vi "extract and prune to time range 3d.vi"(7 "prune?":bool=TRUE, 8 "error in (no error)":errorcluster, 9 "t0":dbl=-1.0, 10 "time range":dbl=-1.0, 11 "queue in":refnum<queue>) -> (0 "error out":errorcluster, 2 "extracted data":T1[](array[typedef]), 3 "queue out":refnum<queue>)   [LabVIEW 2017]
uses:
  typedefs/reading3.ctl
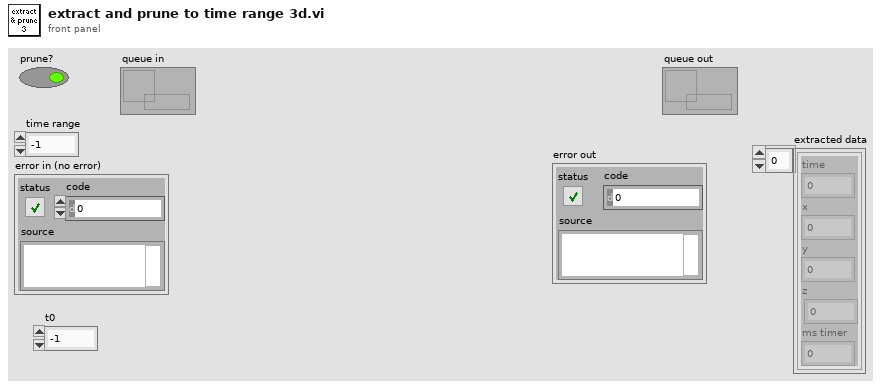
[diagram p1: front panel]
types:
  T1 = typedef "reading3.ctl" = cluster{"time":dbl, "x":dbl, "y":dbl, "z":dbl, "ms timer":u32}
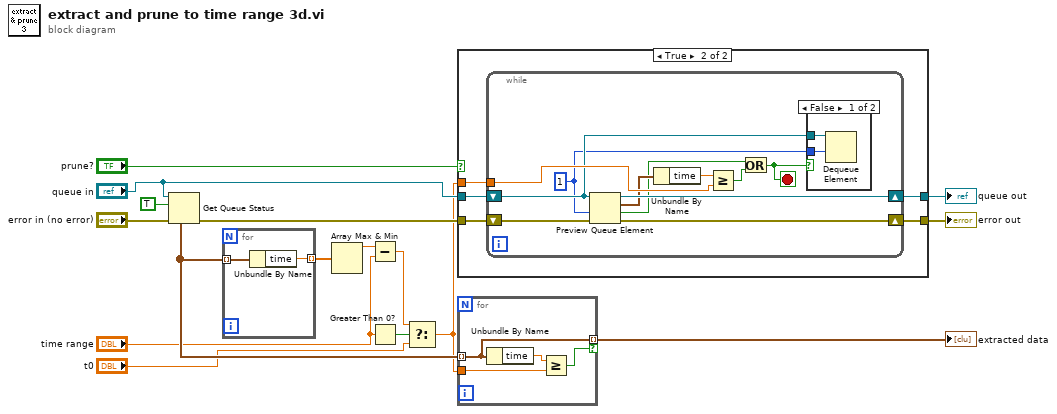
[diagram p0: block diagram]
diagram:
  n1 = Get Queue Status(queue="queue in", return elements? (F)=TRUE, error in (no error)="error in (no error)") -> (error out=w15:errorcluster, elements=w13:T1[])  [unwired: 6 out]
  n2 = for {
    tunnel: w13 -> [w18] mode=indexing
    tunnel: [w17] -> w14 mode=indexing
    n3 = Unbundle By Name(w18) -> ("time"=w17:dbl)
  }
  n4 = Array Max & Min(array=w14) -> (max value=w1:dbl)  [unwired: 3 out]
  n5 = Subtract(x=w1, y="time range") -> (x-y=w4:dbl)
  n6 = Greater Than 0?(x="time range") -> (x > 0?=w6:bool)
  n7 = Select(t=w4, s=w6, f="t0") -> (s? t:f=w3:dbl)
  n8 = case shown="True" "prune?" {
    tunnel: w15 -> [w20 w25]
    tunnel: [w20 w24] -> w11
    tunnel: [w19 w23] -> w10
    tunnel: "queue in" -> [w19 w22]
    tunnel: w3 -> [_ w21]
    frame False {
    }
    frame True {
      n9 = while {
        tunnel: w21 -> [w33]
        shift-right: [w31] -> w24
        shift-left: w25 -> [w36]
        shift-right: [w35] -> w23
        shift-left: w22 -> [w29]
        stop <- w27 stop-if-true
        w28 = 1 ("timeout in ms (-1)")
        n10 = Preview Queue Element(queue=w29, timeout in ms (-1)=w28, error in (no error)=w36) -> (queue out=w35:refnum<queue>, element=w32:T1, timed out?=w26:bool, error out=w31:errorcluster)
        n11 = Unbundle By Name(w32) -> ("time"=w34:dbl)
        n12 = Greater Or Equal?(x=w34, y=w33) -> (x >= y?=w30:bool)
        n13 = Or(x=w26, y=w30) -> (x .or. y?=w27:bool)
        n14 = case shown="False" w27 {
          tunnel: w29 -> [w38 _]
          tunnel: w28 -> [w37 _]
          frame False {
            n15 = Dequeue Element(queue=w38, timeout in ms (-1)=w37) -> ()  [unwired: 1 in, 4 out]
          }
          frame True {
          }
        }
      }
    }
  }
  "error out" <- w11
  "queue out" <- w10
  n16 = for {
    tunnel: w13 -> [w39] mode=indexing
    tunnel: [w39] -> w8 mode=indexing if=w40
    tunnel: w3 -> [w41]
    n17 = Unbundle By Name(w39) -> ("time"=w42:dbl)
    n18 = Greater Or Equal?(x=w42, y=w41) -> (x >= y?=w40:bool)
  }
  "extracted data" <- w8
